vi "example_llm_openaiembedding_unit_test_1.vi"() -> ()   [LabVIEW 2020]
uses:
  src/models/message_vectors/embedding.ctl
  src/models/llm_openai_embedding/llm_openai_embedding.lvclass
  src/models/message_text/message_text.lvclass
  D:/petwork/labview-llm-libraries/src/models/abstract_message_base/abstract_message_base.lvclass
  src/models/message_vectors/message_vectors.lvclass
  src/models/message_text/create_text_message.vi
  src/models/message_vectors/get_vector_message_value.vi
  D:/petwork/labview-llm-libraries/src/models/message_vectors/message_vectors.lvclass
panel:
  out "property:embedding_data":T1[](array[typedef])
  in  "Text":string[](array[string])=["Hello Pineapple", "LLM embedding is not a", "This is not a Rocket Science"]
  out "error out":errorcluster
  out "openai_key":string
  in  "model_name":string(combo)="text-embedding-ada-002"
  # "1. Ensure you assign the OpenAI Key to environmental variables so it is away from the code and easy to use the examples in future.\n\n2. Use the \"Set_ENv_Var.vi\" from examples/utils folder to set the key \"labview_llm_openai_key\"."
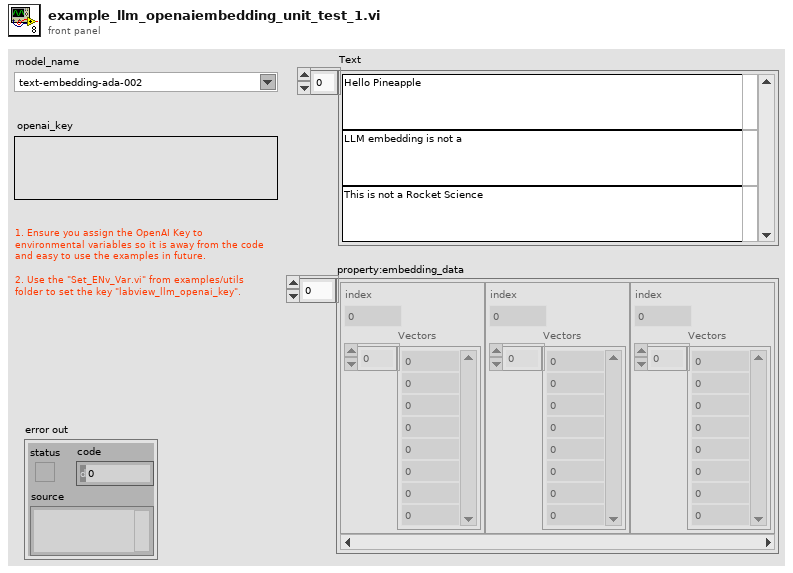
[diagram p1: front panel]
types:
  T1 = typedef "message_vectors.lvclass/embedding.ctl" = cluster{"index":u32, "Vectors":dbl[]}
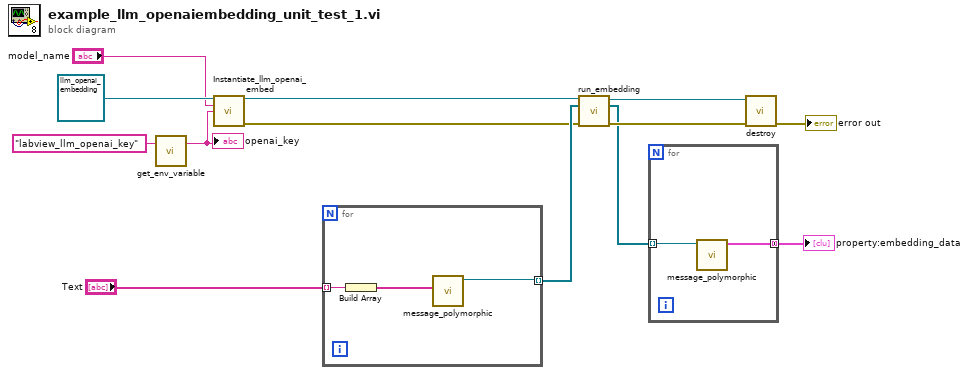
[diagram p0: block diagram]
diagram:
  n1 = call "get_env_variable.vi"("Environment Variable Name"="labview_llm_openai_key") -> ("Value"=w3:string)  [unwired: 1 in, 1 out]
  "openai_key" <- w3
  n2 = call "Instantiate_llm_openai_embed.vi"("llm_openai_embedding in"=refnum<class "llm_openai_embedding.lvclass"> refnum ("llm_openai in"), "model_name"="model_name", "openai_key"=w3) -> ("llm_openai_embedding out"=w13:refnum<class "llm_openai_embedding.lvclass">, "error out"=w5:errorcluster)  [unwired: 11 in]
  n3 = for {
    tunnel: "Text" -> [w16] mode=indexing
    tunnel: [w14] -> w7 mode=indexing
    n4 = Build Array(w16) -> (w15:string[])
    n5 = call-poly "message_polymorphic.vi"("content"=w15) -> ("message_text out"=w14:refnum<class "message_text.lvclass">)  [unwired: 9 in, 1 out]
  }
  n6 = call-dynamic "run_embedding.vi"("llm_openai_embedding in"=w13, "data"=w7, "error in (no error)"=w5) -> ("llm_openai_embedding out"=w11:refnum<class "llm_openai_embedding.lvclass">, "embedding response"=w2:refnum<class "message_vectors.lvclass">[], "error out"=w10:errorcluster)  [unwired: 10 in]
  n7 = for {
    tunnel: [w17] -> w1 mode=concatenating
    tunnel: w2 -> [w18] mode=indexing
    n8 = call-poly "message_polymorphic.vi"("message_vectors in"=w18) -> ("embedding_data"=w17:T1[])  [unwired: 9 in, 1 out]
  }
  "property:embedding_data" <- w1
  n9 = call-dynamic "destroy.vi"("error in (no error)"=w10, "llm_openai_embedding in"=w11) -> ("error out"=→"error out":errorcluster)  [unwired: 8 in, 1 out]
